vi "Refill.vi"(0 "object in":refnum<class "CetoniPump.lvclass">, 2 "index":i32, 5 "error in (no error)":errorcluster) -> (14 "object out":refnum<class "CetoniPump.lvclass">, 19 "error out":errorcluster)   [LabVIEW 2023, in "CetoniPump.lvclass"]
uses:
  CetoniPump.lvclass
  CetoniPump.lvclass/CetoniPump.ctl
  CETONI_SDK/lib/labview/labbCAN_Pump_API/labbCAN_Pump_API.lvlib
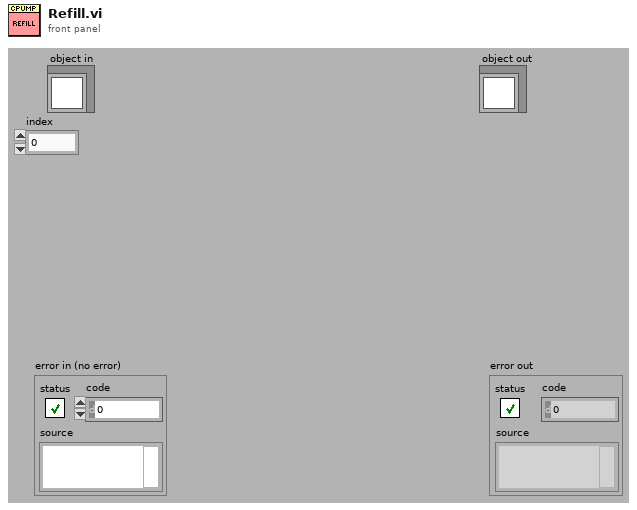
[diagram p1: front panel]
types:
  T1 = cluster{"Pump Handle":i64, "Pump Name":string, "Maximum Volume":dbl, "Maximum Flow Rate":dbl, "Flow Rate":dbl, "Target Level":dbl, "Valve Handle":i64, "Has Valve?":bool, "Actual valve position":i32}[]
  T2 = cluster{"Pump Handle":i64, "Pump Name":string, "Maximum Volume":dbl, "Maximum Flow Rate":dbl, "Flow Rate":dbl, "Target Level":dbl, "Valve Handle":i64, "Has Valve?":bool, "Actual valve position":i32}
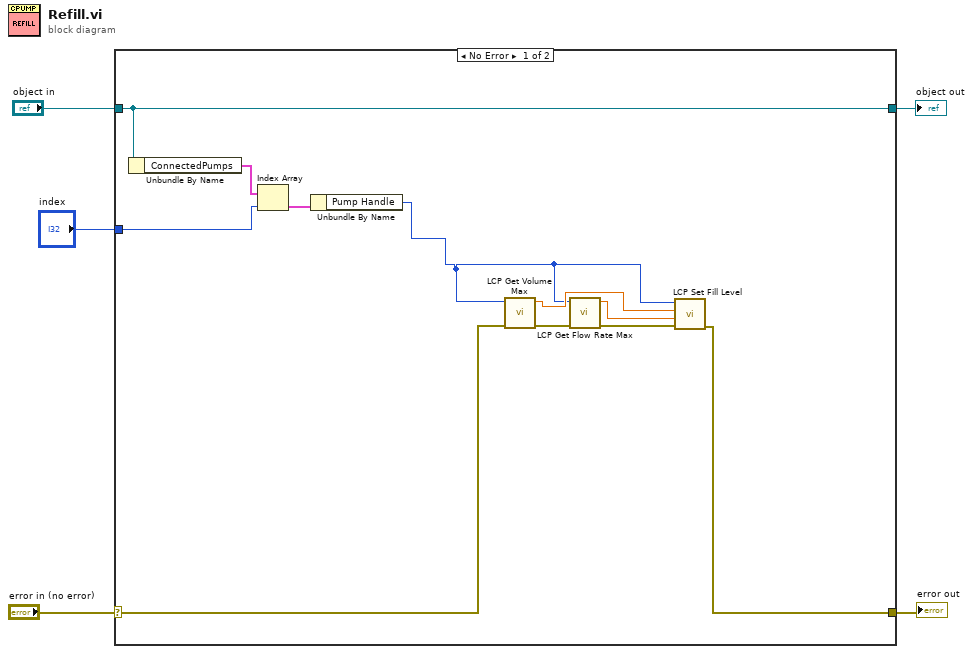
[diagram p0: block diagram]
diagram:
  n1 = case shown="No Error" "error in (no error)" {
    selector: "error in (no error)" -> [w11 w18]
    tunnel: [w10 w18] -> w4
    tunnel: [w16 w17] -> w2
    tunnel: "object in" -> [w16 w17]
    tunnel: "index" -> [w6 _]
    frame No Error {
      n2 = Unbundle By Name(w16) -> ("ConnectedPumps"=w9:T1)
      n3 = Index Array(array=w9, index=w6) -> (element=w8:T2)
      n4 = Unbundle By Name(w8) -> ("Pump Handle"=w7:i64)
      n5 = call "LCP Get Volume Max.vi"("error in (no error)"=w11, "Pump Handle"=w7) -> ("error out"=w15:errorcluster, "Maximum Volume"=w12:dbl)  [unwired: 8 in]
      n6 = call "LCP Get Flow Rate Max.vi"("error in (no error)"=w15, "Pump Handle"=w7) -> ("error out"=w14:errorcluster, "Maximum Flow Rate"=w13:dbl)  [unwired: 8 in]
      n7 = call "LCP Set Fill Level.vi"("error in (no error)"=w14, "Flow"=w13, "Level"=w12, "Pump Handle"=w7) -> ("error out"=w10:errorcluster)  [unwired: 7 in]
    }
    frame Error {
    }
  }
  "error out" <- w4
  "object out" <- w2
